vi "TestLightfieldSettings.vi"() -> ()   [LabVIEW 2018]
uses:
  LightField Automation.lvclass
panel:
  in  "On CCD Accumulations":i32=3 min=0 step=1
  in  "MODE":u16(ring) items=["Normal", "DIF"]
  in  "BIN":u16(ring) items=["1x1", "2x2", "4x4"]
  in  "Number of Frames":i32=500 min=0 step=1
  in  "stop":bool
  out "LightField Error":errorcluster
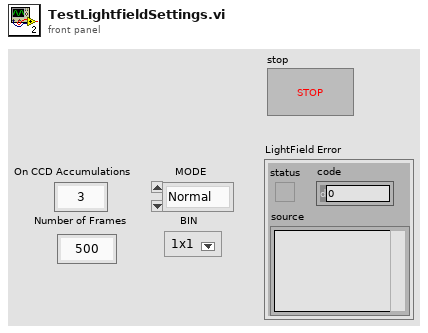
[diagram p1: front panel]
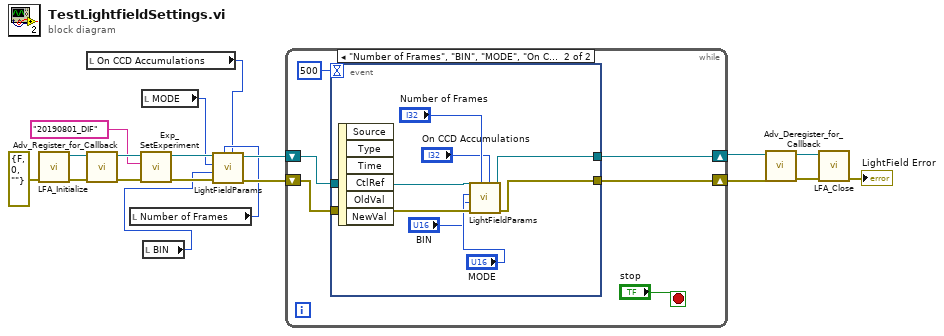
[diagram p0: block diagram]
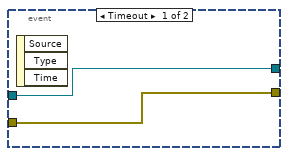
[diagram p2: hidden frame]
diagram:
  n1 = call "LFA_Initialize.vi"("error in (no error)"=errorcluster {"status"=FALSE, "code"=0, "source"=""}) -> ("error out"=w19:errorcluster, "LightField Automation out"=w18:refnum<class "LightField Automation.lvclass">)  [unwired: 9 in]
  n2 = local read "On CCD Accumulations"() -> (w3:i32)
  n3 = call "Adv_Register_for_Callback.vi"("error in (no error)"=w19, "LightField Automation in"=w18) -> ("error out"=w17:errorcluster, "LightField Automation out"=w16:refnum<class "LightField Automation.lvclass">)  [unwired: 8 in]
  n4 = local read "Number of Frames"() -> (w5:i32)
  n5 = call "Exp_SetExperiment.vi"("error in (no error)"=w17, "ExperimentName"="20190801_DIF", "LightField Automation in"=w16) -> ("error out"=w10:errorcluster, "LightField Automation out"=w9:refnum<class "LightField Automation.lvclass">)  [unwired: 7 in]
  n6 = local read "MODE"() -> (w6:u16)
  n7 = local read "BIN"() -> (w4:u16)
  n8 = call "LightFieldParams.vi"("On CCD Accumulations"=w3, "Number of Frames"=w5, "error in"=w10, "BIN"=w4, "MODE"=w6, "LightField Automation in"=w9) -> ("error out"=w7:errorcluster, "LightField Automation out"=w8:refnum<class "LightField Automation.lvclass">)  [unwired: 4 in]
  n9 = while {
    shift-right: [w20] -> w2
    shift-left: w8 -> [w21]
    shift-right: [w22] -> w1
    shift-left: w7 -> [w23]
    stop <- "stop" stop-if-true
    n10 = event shown="[1] \"Number of Frames\", \"BIN\", \"MODE\", \"On CCD Accumulations\": Value Change" {
      selector: _ -> [_ _]
      dyn-events: _ -> [_ _]
      timeout: 500 -> [_ _]
      tunnel: w23 -> [w26 w35]
      tunnel: [w26 w34] -> w22
      tunnel: w21 -> [w27 w33]
      tunnel: [w27 w32] -> w20
      event Timeout {
        n11 = event-data() -> ()  [unwired: 1 in, 3 out]
      }
      event "Number of Frames", "BIN", "MODE", "On CCD Accumulations": Value Change {
        n12 = event-data() -> ()  [unwired: 1 in, 6 out]
        n13 = call "LightFieldParams.vi"("On CCD Accumulations"="On CCD Accumulations", "Number of Frames"="Number of Frames", "error in"=w35, "BIN"="BIN", "MODE"="MODE", "LightField Automation in"=w33) -> ("error out"=w34:errorcluster, "LightField Automation out"=w32:refnum<class "LightField Automation.lvclass">)  [unwired: 4 in]
      }
    }
  }
  n14 = call "Adv_Deregister_for_Callback.vi"("error in (no error)"=w1, "LightField Automation in"=w2) -> ("error out"=w12:errorcluster, "LightField Automation out"=w13:refnum<class "LightField Automation.lvclass">)  [unwired: 8 in]
  n15 = call "LFA_Close.vi"("error in (no error)"=w12, "LightField Automation in"=w13) -> ("error out"=→"LightField Error":errorcluster)  [unwired: 8 in, 1 out]
